vi "TreeView.vi"(7 "Item Indent":i32, 8 "error in (no error)":errorcluster, 10 "Item Reference in":T2 format="%.0x", 11 "Items in":T1(array[cluster])) -> (0 "error out":errorcluster, 3 "Items out":T1(array[cluster]))   [LabVIEW 2013]
uses:
  Item/Ctls/Item Reference.ctl
  Section/Section.lvclass
  Item/Item.lvclass
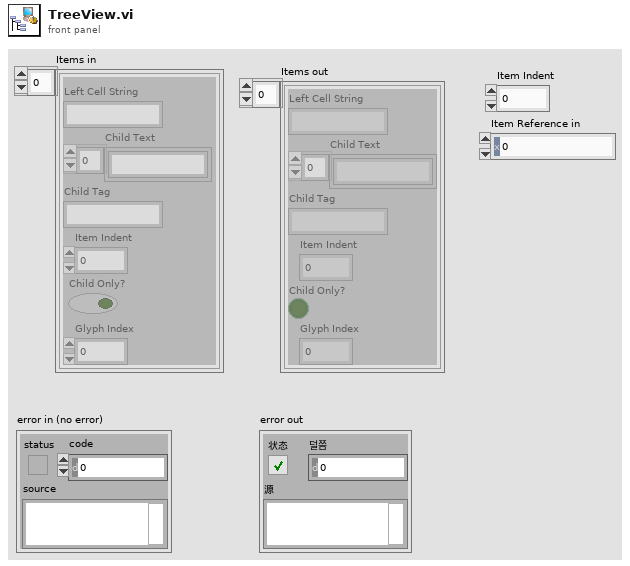
[diagram p1: front panel]
types:
  T1 = cluster{"Left Cell String":string, "Child Text":string[], "Child Tag":string, "Item Indent":i32, "Child Only?":bool, "Glyph Index":i32}[]
  T2 = typedef "Hierarchy Framework.lvlib/Item.lvclass/Item Reference.ctl" = u64
  T3 = cluster{"Left Cell String":string, "Child Text":string[], "Child Tag":string, "Item Indent":i32, "Child Only?":bool, "Glyph Index":i32}
  T4 = typedef "Hierarchy Framework.lvlib/Item.lvclass/Item Info.ctl" = cluster{"Name":string, "TagGUID":string, "TypeGUID":string, "Enable":bool}
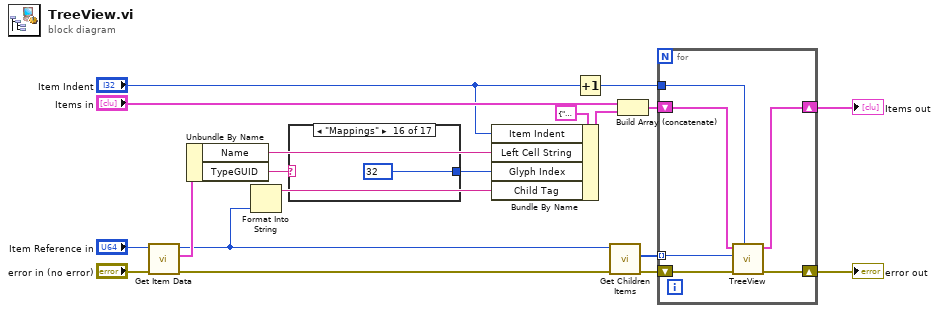
[diagram p0: block diagram]
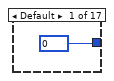
[diagram p2: hidden frame]
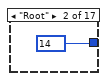
[diagram p3: hidden frame]
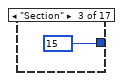
[diagram p4: hidden frame]
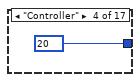
[diagram p5: hidden frame]
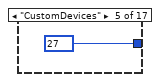
[diagram p6: hidden frame]
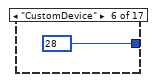
[diagram p7: hidden frame]
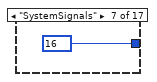
[diagram p8: hidden frame]
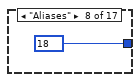
[diagram p9: hidden frame]
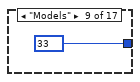
[diagram p10: hidden frame]
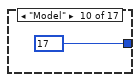
[diagram p11: hidden frame]
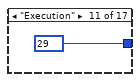
[diagram p12: hidden frame]
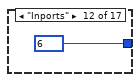
[diagram p13: hidden frame]
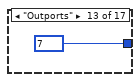
[diagram p14: hidden frame]
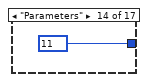
[diagram p15: hidden frame]
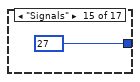
[diagram p16: hidden frame]
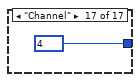
[diagram p17: hidden frame]
diagram:
  n1 = call "Get Item Data.vi"("error in (no error)"="error in (no error)", "Item Reference in"="Item Reference in") -> ("error out"=w18:errorcluster, "Item Info"=w17:T4, "Item Reference out"=w2:T2)  [unwired: 6 in, 1 out]
  n2 = Unbundle By Name(w17) -> ("Name"=w16:string, "TypeGUID"=w5:string)
  n3 = Format Into String(w2) -> (resulting string=w1:string)  [unwired: 3 in, 1 out]
  n4 = case shown="\"Mappings\"" w5 {
    tunnel: [0 14 15 20 27 28 16 18 33 17 29 6 7 11 27 32 4] -> w4
    frame Default {
    }
    frame "Root" {
    }
    frame "Section" {
    }
    frame "Controller" {
    }
    frame "CustomDevices" {
    }
    frame "CustomDevice" {
    }
    frame "SystemSignals" {
    }
    frame "Aliases" {
    }
    frame "Models" {
    }
    frame "Model" {
    }
    frame "Execution" {
    }
    frame "Inports" {
    }
    frame "Outports" {
    }
    frame "Parameters" {
    }
    frame "Signals" {
    }
    frame "Mappings" {
    }
    frame "Channel" {
    }
  }
  n5 = Bundle By Name(cluster=T3 {"Left Cell String"="", "Child Text"=[], "Child Tag"="", "Item Indent"=0, "Child Only?"=FALSE, "Glyph Index"=0} ("Item"), "Item Indent"="Item Indent", "Left Cell String"=w16, "Glyph Index"=w4, "Child Tag"=w1) -> (w15:T3)
  n6 = Increment(x="Item Indent") -> (x+1=w9:i32)
  n7 = call "Get Children Items.vi"("error in (no error)"=w18, "Section Reference in"=w2) -> ("error out"=w7:errorcluster, "Children Item References"=w19:u64[])  [unwired: 5 in, 3 out]
  n8 = Build Array (concatenate)("Items in", w15) -> (w14:T1)
  n9 = for {
    tunnel: w19 -> [w37] mode=indexing
    shift-right: [w40] -> w8
    shift-left: w14 -> [w42]
    tunnel: w9 -> [w38]
    shift-right: [w39] -> w6
    shift-left: w7 -> [w41]
    n10 = call "TreeView.vi"("Item Indent"=w38, "error in (no error)"=w41, "Item Reference in"=w37, "Items in"=w42) -> ("error out"=w39:errorcluster, "Items out"=w40:T1)  [unwired: 6 in]
  }
  "Items out" <- w8
  "error out" <- w6
